vi "Get Monotonically Increasing State Value.vi"(8 "error in (no error)":errorcluster, 10 "State Values":i32[](array[numeric]), 11 "Desire State Value":i32) -> (0 "error out":errorcluster, 3 "New State Value":i32)   [LabVIEW 2020, in "Routing and Faulting System Explorer.lvlib"]
uses:
  Routing and Faulting System Explorer.lvlib
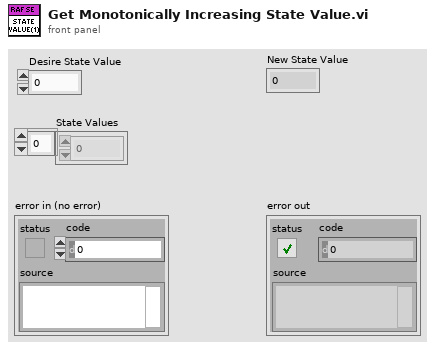
[diagram p1: front panel]
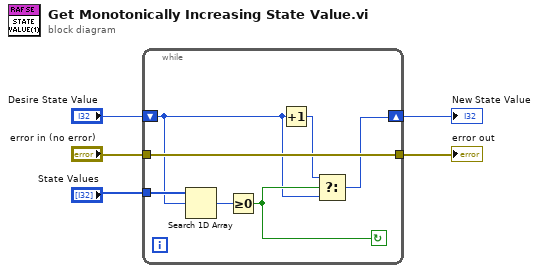
[diagram p0: block diagram]
diagram:
  n1 = while {
    tunnel: "error in (no error)" -> [w12]
    shift-right: [w8] -> w1
    shift-left: "Desire State Value" -> [w6]
    tunnel: [w12] -> w3
    tunnel: "State Values" -> [w10]
    stop <- w9 continue-if-true
    n2 = Search 1D Array(1D array=w10, element=w6) -> (index of element=w11:i32)  [unwired: 1 in]
    n3 = Greater Or Equal To 0?(x=w11) -> (x >= 0?=w9:bool)
    n4 = Increment(x=w6) -> (x+1=w7:i32)
    n5 = Select(t=w7, s=w9, f=w6) -> (s? t:f=w8:i32)
  }
  "New State Value" <- w1
  "error out" <- w3
